vi "I2C Operation_old.vi"(6 "input_data":u8[](array[numeric]) format="%.0x", 7 "size":i32, 8 "Channel":u8 max=5 step=1, 9 "address":u8, 10 "mode":string(combo)="read", 11 "VISA":refnum<visa-resource-name>="COM6") -> (1 "result":bool, 2 "message":string, 3 "Data Out":u8[](array[numeric]) format="%.0x")   [LabVIEW 2011]
panel:
  out "无符号字节数组":u8[](array[numeric]) format="%.0x"
  out "write error":string
  out "read error":u8[](array[numeric]) format="%.0x"
  # "0"
  # "1"
  # "2"
  # "3"
  # "4"
  # "5"
  # "6"
  # "7"
  # "8"
  # "9"
  # "10"
  # "11"
  # "12"
  # "13"
  # "14"
  # "15"
  # "16"
  # "17"
  # "18"
  # "19"
  # "20"
  # "21"
  # "I2C EEPROM Opertion"
  # "10"
  # "0"
  # "5"
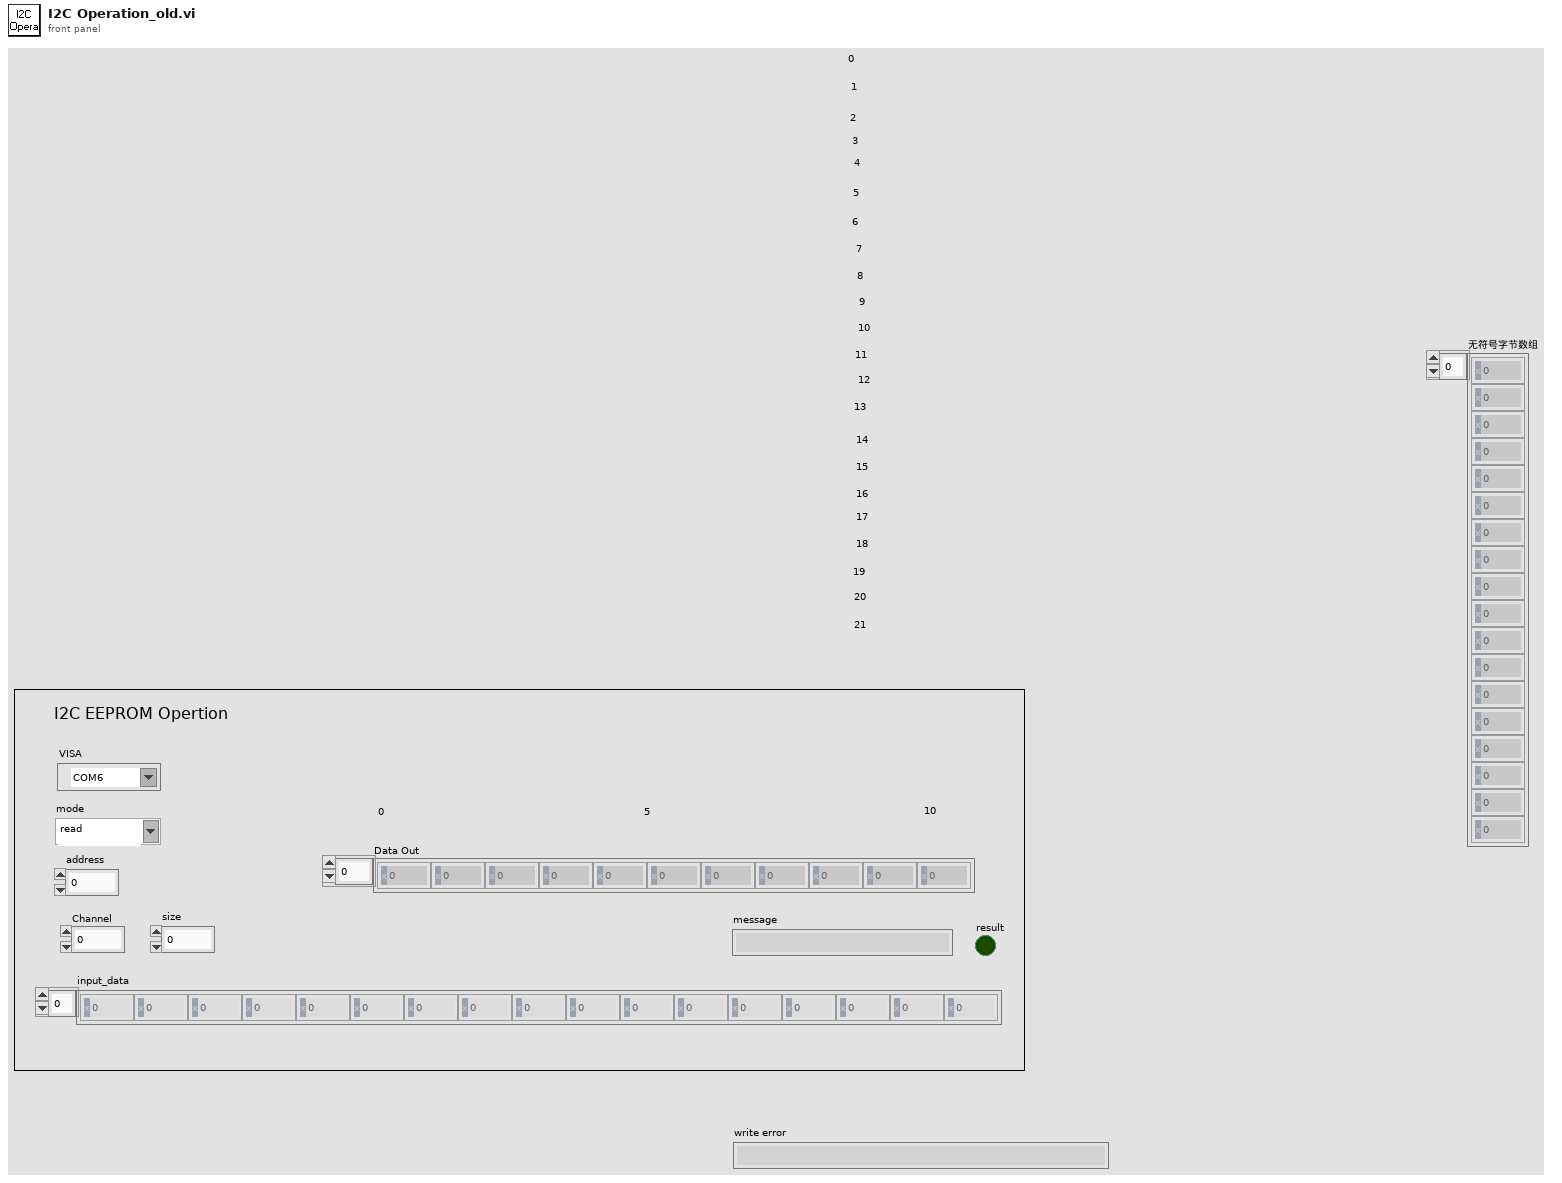
[diagram p1: front panel]
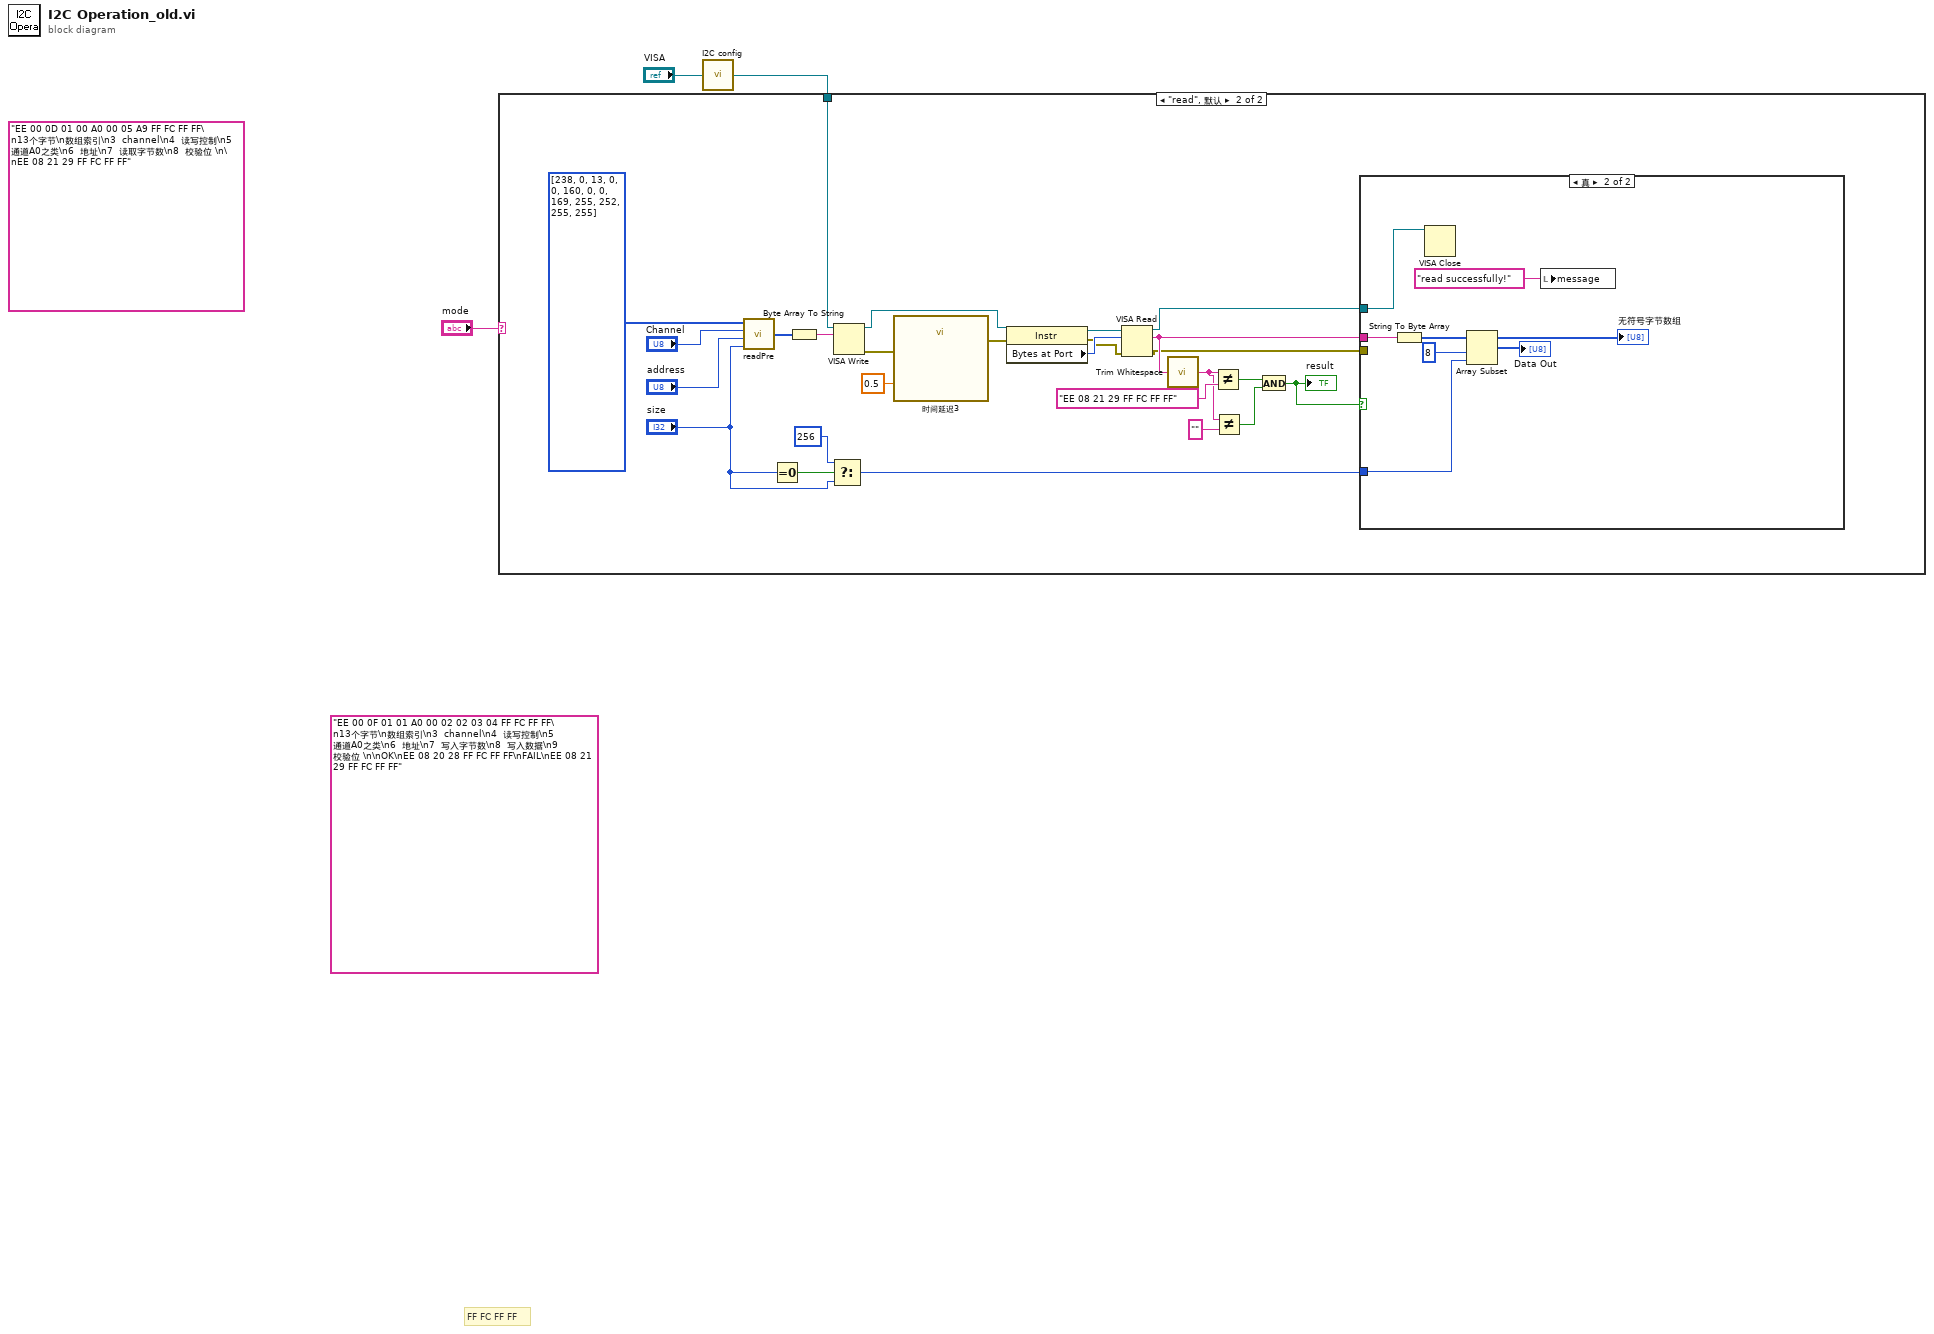
[diagram p0: block diagram]
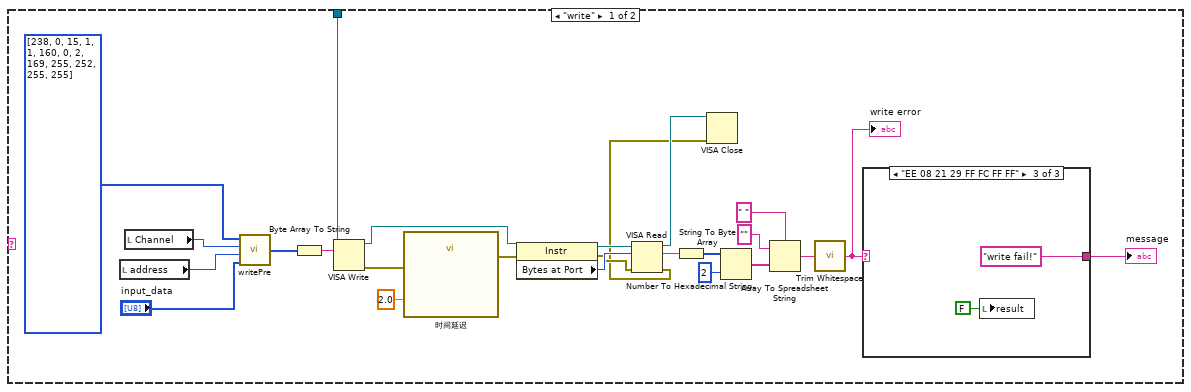
[diagram p2: hidden frame]
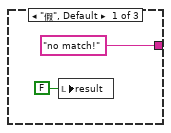
[diagram p3: hidden frame]
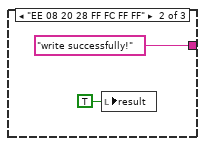
[diagram p4: hidden frame]
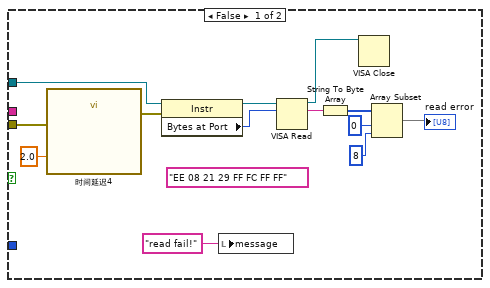
[diagram p5: hidden frame]
diagram:
  (unwired) "EE 00 0F 01 01 A0 00 02 02 03 04 FF FC FF FF\n13个字节\n数组索引\n3  channel\n4  读写控制\n5  通道A0之类\n6  地址\n7  写入字节数\n8  写入数据\n9  校验位 \n\nOK\nEE 08 20 28 FF FC FF FF\nFAIL\nEE 08 21 29 FF FC FF FF"
  (unwired) "EE 00 0D 01 00 A0 00 05 A9 FF FC FF FF\n13个字节\n数组索引\n3  channel\n4  读写控制\n5  通道A0之类\n6  地址\n7  读取字节数\n8  校验位 \n\nEE 08 21 29 FF FC FF FF"
  # "FF FC FF FF"
  n1 = call "I2C config.vi"("VISA"="VISA") -> ("VISA资源名称输出"=w2:refnum<visa-resource-name>)
  n2 = case shown="\"read\", 默认" "mode" {
    tunnel: w2 -> [w25 w57]
    frame "write" {
      n3 = local read "address"() -> (w17:u8)
      n4 = local read "Channel"() -> (w18:u8)
      n5 = call "writePre.vi"("input_data"="input_data", "address"=w17, "Channel"=w18, "order"=u8[] [238, 0, 15, 1, 1, 160, 0, 2, 169, 255, 252, 255, 255]) -> ("out"=w14:u8[])
      n6 = Byte Array To String(unsigned byte array=w14) -> (string=w28:string)
      n7 = VISA Write(VISA resource name=w25, write buffer=w28) -> (VISA resource name out=w20:refnum<visa-resource-name>, error out=w24:errorcluster)  [unwired: 1 in, 1 out]
      n8 = call "时间延迟"("error in (no error)"=w24, "Delay Time (s)"=2.0) -> ("error out"=w23:errorcluster)  [unwired: 9 in]
      n9 = property class="Instr"(reference=w20, error in=w23) -> (reference out=w26:refnum<visa-resource-name>, error out=w21:errorcluster, "Bytes at Port"=w27:u32)
      n10 = VISA Read(VISA resource name=w26, byte count=w27, error in (no error)=w21) -> (VISA resource name out=w5:refnum<visa-resource-name>, read buffer=w13:string, error out=w4:errorcluster)  [unwired: 1 out]
      n11 = String To Byte Array(string=w13) -> (unsigned byte array=w12:u8[])
      n12 = VISA Close(VISA resource name=w5, error in (no error)=w4) -> ()  [unwired: 1 out]
      n13 = Number To Hexadecimal String(1:i16 2 ("宽度(-)"), 2:w12) -> (0:w11:string[])
      n14 = Array To Spreadsheet String(delimiter (Tab)=" " ("分隔符(Tab)"), array=w11, 3:"" ("格式字符串")) -> (spreadsheet string=w8:string)
      n15 = call <vilib>:"Trim Whitespace.vi"("string"=w8) -> ("trimmed string"=w6:string)  [unwired: 1 in]
      "write error" <- w6
      n16 = case shown="\"EE 08 21 29 FF FC FF FF\"" w6 {
        tunnel: ["no match!" "write successfully!" "write fail!"] -> w19
        frame "假", Default {
          n17 = local write "result"(FALSE ("result")) -> ()
        }
        frame "EE 08 20 28 FF FC FF FF" {
          n18 = local write "result"(TRUE ("result")) -> ()
        }
        frame "EE 08 21 29 FF FC FF FF" {
          n19 = local write "result"(FALSE ("result")) -> ()
        }
      }
      "message" <- w19
    }
    frame "read", Default {
      n20 = call "readPre.vi"("size"="size", "address"="address", "Channel"="Channel", "input_order"=u8[] [238, 0, 13, 0, 0, 160, 0, 0, 169, 255, 252, 255, 255]) -> ("out"=w40:u8[])
      n21 = Equal To 0?(x="size") -> (x = 0?=w38:bool)
      n22 = Byte Array To String(unsigned byte array=w40) -> (string=w60:string)
      n23 = Select(t=256, s=w38, f="size") -> (s? t:f=w37:i32)
      n24 = VISA Write(VISA resource name=w57, write buffer=w60) -> (VISA resource name out=w44:refnum<visa-resource-name>, error out=w56:errorcluster)  [unwired: 1 in, 1 out]
      n25 = call "时间延迟3"("error in (no error)"=w56, "Delay Time (s)"=0.5) -> ("error out"=w55:errorcluster)  [unwired: 9 in]
      n26 = property class="Instr"(reference=w44, error in=w55) -> (reference out=w58:refnum<visa-resource-name>, error out=w46:errorcluster, "Bytes at Port"=w59:u32)
      n27 = VISA Read(VISA resource name=w58, byte count=w59, error in (no error)=w46) -> (VISA resource name out=w39:refnum<visa-resource-name>, read buffer=w47:string, error out=w45:errorcluster)  [unwired: 1 out]
      n28 = call <vilib>:"Trim Whitespace.vi"("string"=w47) -> ("trimmed string"=w52:string)  [unwired: 1 in]
      n29 = Not Equal?(x=w52, y="EE 08 21 29 FF FC FF FF") -> (x != y?=w50:bool)
      n30 = Not Equal?(x=w52, y="") -> (x != y?=w49:bool)
      n31 = And(x=w50, y=w49) -> (x .and. y?=w48:bool)
      "result" <- w48
      n32 = case shown="真" w48 {
        tunnel: w47 -> [_ w77]
        tunnel: w39 -> [w69 w75]
        tunnel: w45 -> [w68 _]
        tunnel: w37 -> [_ w74]
        frame False {
          (unwired) "EE 08 21 29 FF FC FF FF"
          n33 = call "时间延迟4"("error in (no error)"=w68, "Delay Time (s)"=2.0) -> ("error out"=w71:errorcluster)  [unwired: 9 in]
          n34 = property class="Instr"(reference=w69, error in=w71) -> (reference out=w72:refnum<visa-resource-name>, "Bytes at Port"=w73:u32)  [unwired: 1 out]
          n35 = local write "message"("read fail!" ("message")) -> ()
          n36 = VISA Read(VISA resource name=w72, byte count=w73) -> (VISA resource name out=w61:refnum<visa-resource-name>, read buffer=w63:string)  [unwired: 1 in, 2 out]
          n37 = String To Byte Array(string=w63) -> (unsigned byte array=w67:u8[])
          n38 = VISA Close(VISA resource name=w61) -> ()  [unwired: 1 in, 1 out]
          n39 = Array Subset(array=w67, index=0 ("索引"), length=8 ("长度")) -> (→"read error":u8[])
        }
        frame True {
          n40 = String To Byte Array(string=w77) -> (unsigned byte array=w80:u8[])
          "无符号字节数组" <- w80
          n41 = VISA Close(VISA resource name=w75) -> ()  [unwired: 1 in, 1 out]
          n42 = Array Subset(array=w80, index=8 ("索引"), length=w74) -> (→"Data Out":u8[])
          n43 = local write "message"("read successfully!" ("message")) -> ()
        }
      }
    }
  }
